vi "Cleanup.vi"(8 "error in (no error)":errorcluster, 11 "CLI in":refnum<class "CLI.lvclass">) -> (0 "error out":errorcluster)   [LabVIEW 2020, in "neg-pkg-cli.lvlib" / "CLI.lvclass"]
uses:
  CLI.lvclass
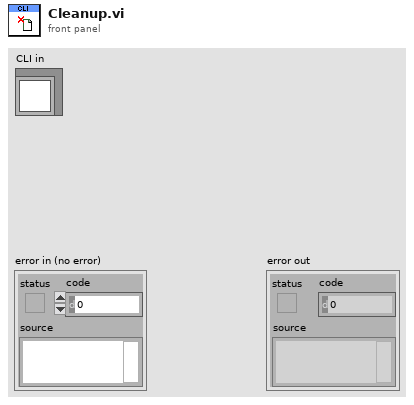
[diagram p1: front panel]
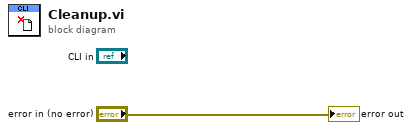
[diagram p0: block diagram]
diagram:
  "error out" <- "error in (no error)"
